vi "prototype UI_RESONANT.vi.REMOTE.vi"() -> ()   [LabVIEW 2012]
uses:
  GFG/GFG library.lvlib
  <vilib>/event_ctls.llb/lveventtype.ctl
  Custom Controls/scan mode main settings tab.ctl
  Custom Controls/file format type def.ctl
  Custom Controls/MAIN Image panel tab Control type def.ctl
  Custom Controls/Ch selector.ctl
  Custom Controls/advanced settings inner tab CTL.ctl
  Custom Controls/pixel resolution enum.ctl
  Custom Controls/display palette control.ctl
  Custom Controls/experiment type.ctl
  Custom Controls/Histogram tab.ctl
panel:
  in  "Objective":u16(ring) items=["10x Olympus", "20x Nikon", "30x Zeiss"]
  in  "x.voltage":dbl=0.9999999999999999 min=0.0 max=5.5 step=0.1
  in  "y.voltage":dbl=1.0 min=0.0 max=5.5 step=0.1
  in  "y.volt.offset":dbl=-0.2 step=0.1
  in  "x.volt.offset":dbl=-0.2 step=0.1
  in  "shutter":bool
  in  "x.pixels":i32=256 min=2 max=2048 step=2
  in  "clear prot":bool
  in  "timestamp.prot":bool
  in  "protocol.notes":string caption="notebook"
  in  "pos \nstore F":bool
  in  "pos \nstore E":bool
  in  "pos \nstore D":bool
  in  "pos \nstore C":bool
  in  "pos \nstore B":bool
  in  "pos \nstore A":bool
  out "String 10":string
  in  "pos \nrecall F":bool
  in  "pos \nrecall E":bool
  in  "pos \nrecall D":bool
  in  "pos \nrecall C":bool
  in  "pos \nrecall B":bool
  in  "pos \nrecall A":bool
  out "String 11":string
  in  "ref img\nOpen Files Button":bool
  in  "ref img\nstore F":bool
  in  "ref img\nstore E":bool
  in  "ref img\nstore D":bool
  in  "ref img\nstore C":bool
  in  "ref img\nstore B":bool
  in  "ref img\nstore A":bool
  out "String 17":string
  in  "ref img\nSave As Button":bool
  in  "Open All\nSettings":bool
  in  "step.size.z":u16(ring)=6 items=["  1"=1, "  2"=2, "  5"=5, " 10"=10, " 20"=20, " 50"=50, "100"=100]
  in  "Stage Stop":bool
  out "frame count":dbl(slide) scale=-1.0..430000.0
  in  "scan mode main settings":T1
  in  "x.correction":dbl(slide)=30.0 min=-100.0 max=100.0 step=1.0 scale=-100.0..100.0 scale format="%#_3g"
  in  "Start.Delay":dbl(slide)=220.0 min=1.0 max=320.0 step=1.0 scale=1.0..320.0 scale format="%#_3g"
  in  "pixel resolution":T2
  in  "ZOOM":dbl(slide)=1.0 min=1.0 max=3.0 step=0.1 scale=1.0..3.0 scale format="%_2g"
  in  "no. of frames to acquire":i32=10000 min=2 max=2147483646 step=2
  in  "x.fov":dbl caption="Field of view    x" format="%#_3p"
  in  "y.fov":dbl caption="y" format="%#_3p"
  out "frames.p.sec":dbl caption="frames/s" format="%#.2g"
  in  "resonant.correction.enable":bool
  out "pixels per line":i32=10000 min=2 max=2147483646 step=2
  out "lines per second":i32=10000 min=2 max=2147483646 step=2
  in  "linescan.y.pixels":i32=256 caption="Lines to display at once" min=2 max=2048 step=2
  in  "no. of lines to acquire":i32=10000 min=2 max=2147483646 step=2
  in  "experiment type":T3
  in  "experiment name":string
  in  "root.path":path=path "g:/"
  in  "file format":T4
  out "stack.duration":i32=10 caption="stack.duration (sec)" min=0 max=2147483646 step=2
  out "interpol XY":cluster{dbl[], "Best Exponential Fit":dbl[]}[](graph)
  in  "add":bool
  in  "clear all":bool
  in  "clear last":bool
  in  "move to z.stack.\nstart plane":bool
  in  "start z.stack":bool
  in  "frames.per.plane":i32=10000
  in  "z.spacing":dbl=1.0 caption="z.spacing (um)" min=0.1 step=0.1
  out "no of planes":i32=10 min=0 max=2147483646 step=2
  in  "piezo.mode":bool
  in  "frames.per.z.cycle":dbl=2.0 min=2.0 max=100.0 step=1.0
  in  "piezo.active":bool
  in  "Z UP":bool
  in  "Z DOWN":bool
  out "String 7":string
  in  "step.size.xy":u16(ring)=6 items=["  1"=1, "  2"=2, "  5"=5, " 10"=10, " 20"=20, " 50"=50, "100"=100]
  in  "Y UP":bool
  in  "X LEFT":bool
  in  "Y DOWN":bool
  in  "X RIGHT":bool
  out "String 6":string
  in  "setY":dbl caption="Z-Stepper" format="%#.1f"
  in  "setX":dbl caption="Z-Stepper" format="%#.1f"
  in  "setZ":dbl caption="set" format="%#.1f"
  out "String 4":string
  out "posZ":dbl caption="actual" format="%#.1f"
  out "posX":dbl caption="Z-Stepper" format="%#.1f"
  out "posY":dbl caption="Z-Stepper" format="%#.1f"
  out "String 3":string
  in  "XYZ stage settings slider tab":enum32{" "}(tab)
  in  "set Y to zero":bool
  in  "set X to zero":bool
  in  "set all to zero":bool
  in  "set Z to zero":bool
  out "String 9":string
  in  "reverse y":bool
  in  "reverse x":bool
  in  "reverse z":bool
  out "String 8":string
  in  "PIN Button stage settings":bool
  in  "QUIT":bool
  in  "Record":bool
  in  "FOCUS":bool
  in  "MAIN Image panels":T5
  out "Channel 1 large":T6(plugin-control)
  out "Channel 2 large":T6(plugin-control)
  out "Channel 3 large":T6(plugin-control)
  out "Channel 4 large":T6(plugin-control)
  out "Channel 1 small":T6(plugin-control)
  out "Channel 2 small":T6(plugin-control)
  out "Channel 4 small":T6(plugin-control)
  out "Channel 3 small":T6(plugin-control)
  in  "Blue Channel (Overlay)":T7 caption="B"
  in  "Green Channel (Overlay)":T7=enum."Ch 1" caption="G"
  in  "Red Channel (Overlay)":T7=enum."Ch 2" caption="R"
  out "RGB overlay":T6(plugin-control)
  out "ROI chart":sgl[][](graph)=[[54.570076, 54.556858]]
  in  "ROI channel":T7=enum."Ch 1" caption="Channel"
  out "ROI Image display":T6(plugin-control)
  in  "confirm line":bool
  in  "channel arb line scan":T7 caption="Channel"
  out "arb line scan display":T6(plugin-control)
  in  "Cancel":bool
  in  "hist/ref slider tab":enum32{" "}(tab)
  in  "PIN Button Hist/Ref":bool
  in  "Histograms tab":T8
  in  "auto scale\n      CH 1":bool=TRUE caption="auto scale 2"
  in  "Min Max Channel 1":cluster{dbl, dbl}(slide) scale=-33000.0..33000.0 scale format="%#_5g"
  out "Histogram 1":T9(graph)
  out "String 12":string
  in  "auto scale\n      CH 4":bool=TRUE caption="auto scale 2"
  in  "Min Max Channel 4":cluster{dbl, dbl}(slide) scale=-100.0..2047.0 scale format="%#_4g"
  out "Histogram 4":T9(graph)
  out "String 15":string
  in  "auto scale\n      CH 3":bool=TRUE caption="auto scale 2"
  in  "Min Max Channel 3":cluster{dbl, dbl}(slide) scale=-100.0..2047.0 scale format="%#_4g"
  out "Histogram 3":T9(graph)
  out "String 14":string
  in  "auto scale\n      CH 2":bool=TRUE caption="auto scale 2"
  in  "Min Max Channel 2":cluster{dbl, dbl}(slide) scale=-33000.0..33000.0 scale format="%#_4g"
  out "Histogram 2":T9(graph)
  out "String 13":string
  in  "avg type":u16(ring) items=["none", "group avg", "moving avg"]
  in  "avg of":i8=10 min=2 step=1
  in  "display palette":T10
  in  "laser power slider tab":enum32{""}(tab)
  in  "Laser Power":dbl(knob) min=0.0 max=100.0 step=0.5 scale=0.0..100.0 scale format="%3d"
  in  "PIN Button Pockels Control":bool
  in  "PMT slider tab":enum32{""}(tab)
  in  "PMT 2":u16(slide) max=1000 scale=0.0..1000.0
  in  "PMT 1":u16(slide) max=1250 scale=0.0..1000.0
  out "String 5":string
  in  "PMT 4":u16(slide) max=1000 scale=0.0..1000.0
  in  "PMT 3":u16(slide) max=1250 scale=0.0..1000.0
  out "String 18":string
  in  "PIN Button PMTs":bool
  in  "advanced settings slider tab":enum32{""}(tab)
  in  "advanced settings inner tab":T11
  in  "y.pixel.sz":dbl=1e-05 min=1e-09 max=1e-05 step=1e-07 format="%#_3p"
  in  "x.pixel.sz":dbl=1e-05 min=1e-09 max=1e-05 step=1e-07 format="%#_3p"
  in  "y.pixels":i32=256 caption="Y Resolution" min=2 max=2048 step=2
  in  "nomin.x.pixels":i32=256 caption="X resolution" min=2 max=2048 step=2
  in  "max.field.of.view\nresonant":dbl=300.0 format="%#_6p"
  in  "voltage.for\nmax.field.of.view\nresonant":dbl=5.0
  in  "max.field.of.view":dbl=300.0 format="%#_6p"
  in  "voltage.for\nmax.field.of.view":dbl=5.0
  in  "ai.active3":bool
  in  "ai.active2":bool
  in  "ai.active1":bool
  in  "ai.active0":bool caption="active?"
  in  "ai.range2":dbl=10.0 min=0.1 max=10.0 step=0.1
  in  "ai.range1":dbl=10.0 min=0.1 max=10.0 step=0.1
  out "ai.string3":string
  out "ai.string2":string
  out "ai.string1":string
  out "ai.string0":string caption="Analog Input"
  in  "ai.range0":dbl=10.0 caption="input range" min=0.1 max=10.0 step=0.1
  in  "ai.range3":dbl=10.0 min=0.1 max=10.0 step=0.1
  in  "external.start.trigger.enable":bool=TRUE caption="WAIT FOR TRIGGER"
  in  "pos  pockels cell PMT Data":dbl[][](array[numeric])=[[0.0, 0.0, 0.0, 0.0, 0.0, 0.0], [-200.0, 0.0, 0.0, 0.0, 0.0, 0.0]] caption="Data" format="%0.1f"
  in  "PIN Button Advanced Settings":bool
  in  "SCIENTIFICA Button":bool
  # "to zoom out press and hold Shift"
  # "current pos."
  # "go to pos."
  # "STORE positions"
  # "RECALL  positions"
  # "REFERENCE IMAGES"
  # "STORE"
  # "zig-zag (leaf scan)"
  # "planes"
  # "set zero"
  # "reverse \ndirection"
  # "1"
  # "2"
  # "3"
  # "4"
  # "Press and hold Ctrl to add multiple ROIs"
  # "This checkbox is only for starting the image acquisition using a TTL rising edge trigger from an external device. Don't tick this box unless an incoming trigger is wired up, otherwise the software may freeze. To reset, click QUIT and restart. If you want to send a trigger to an external device, just connect the ai.start.trigger.channel (e.g.PFI2, specified in settings.INI) to the external device, but leave the  checkbox above unticked."
  # "Z"
  # "laser"
  # "PMT1"
  # "PMT2"
  # "PMT3"
  # "PMT4"
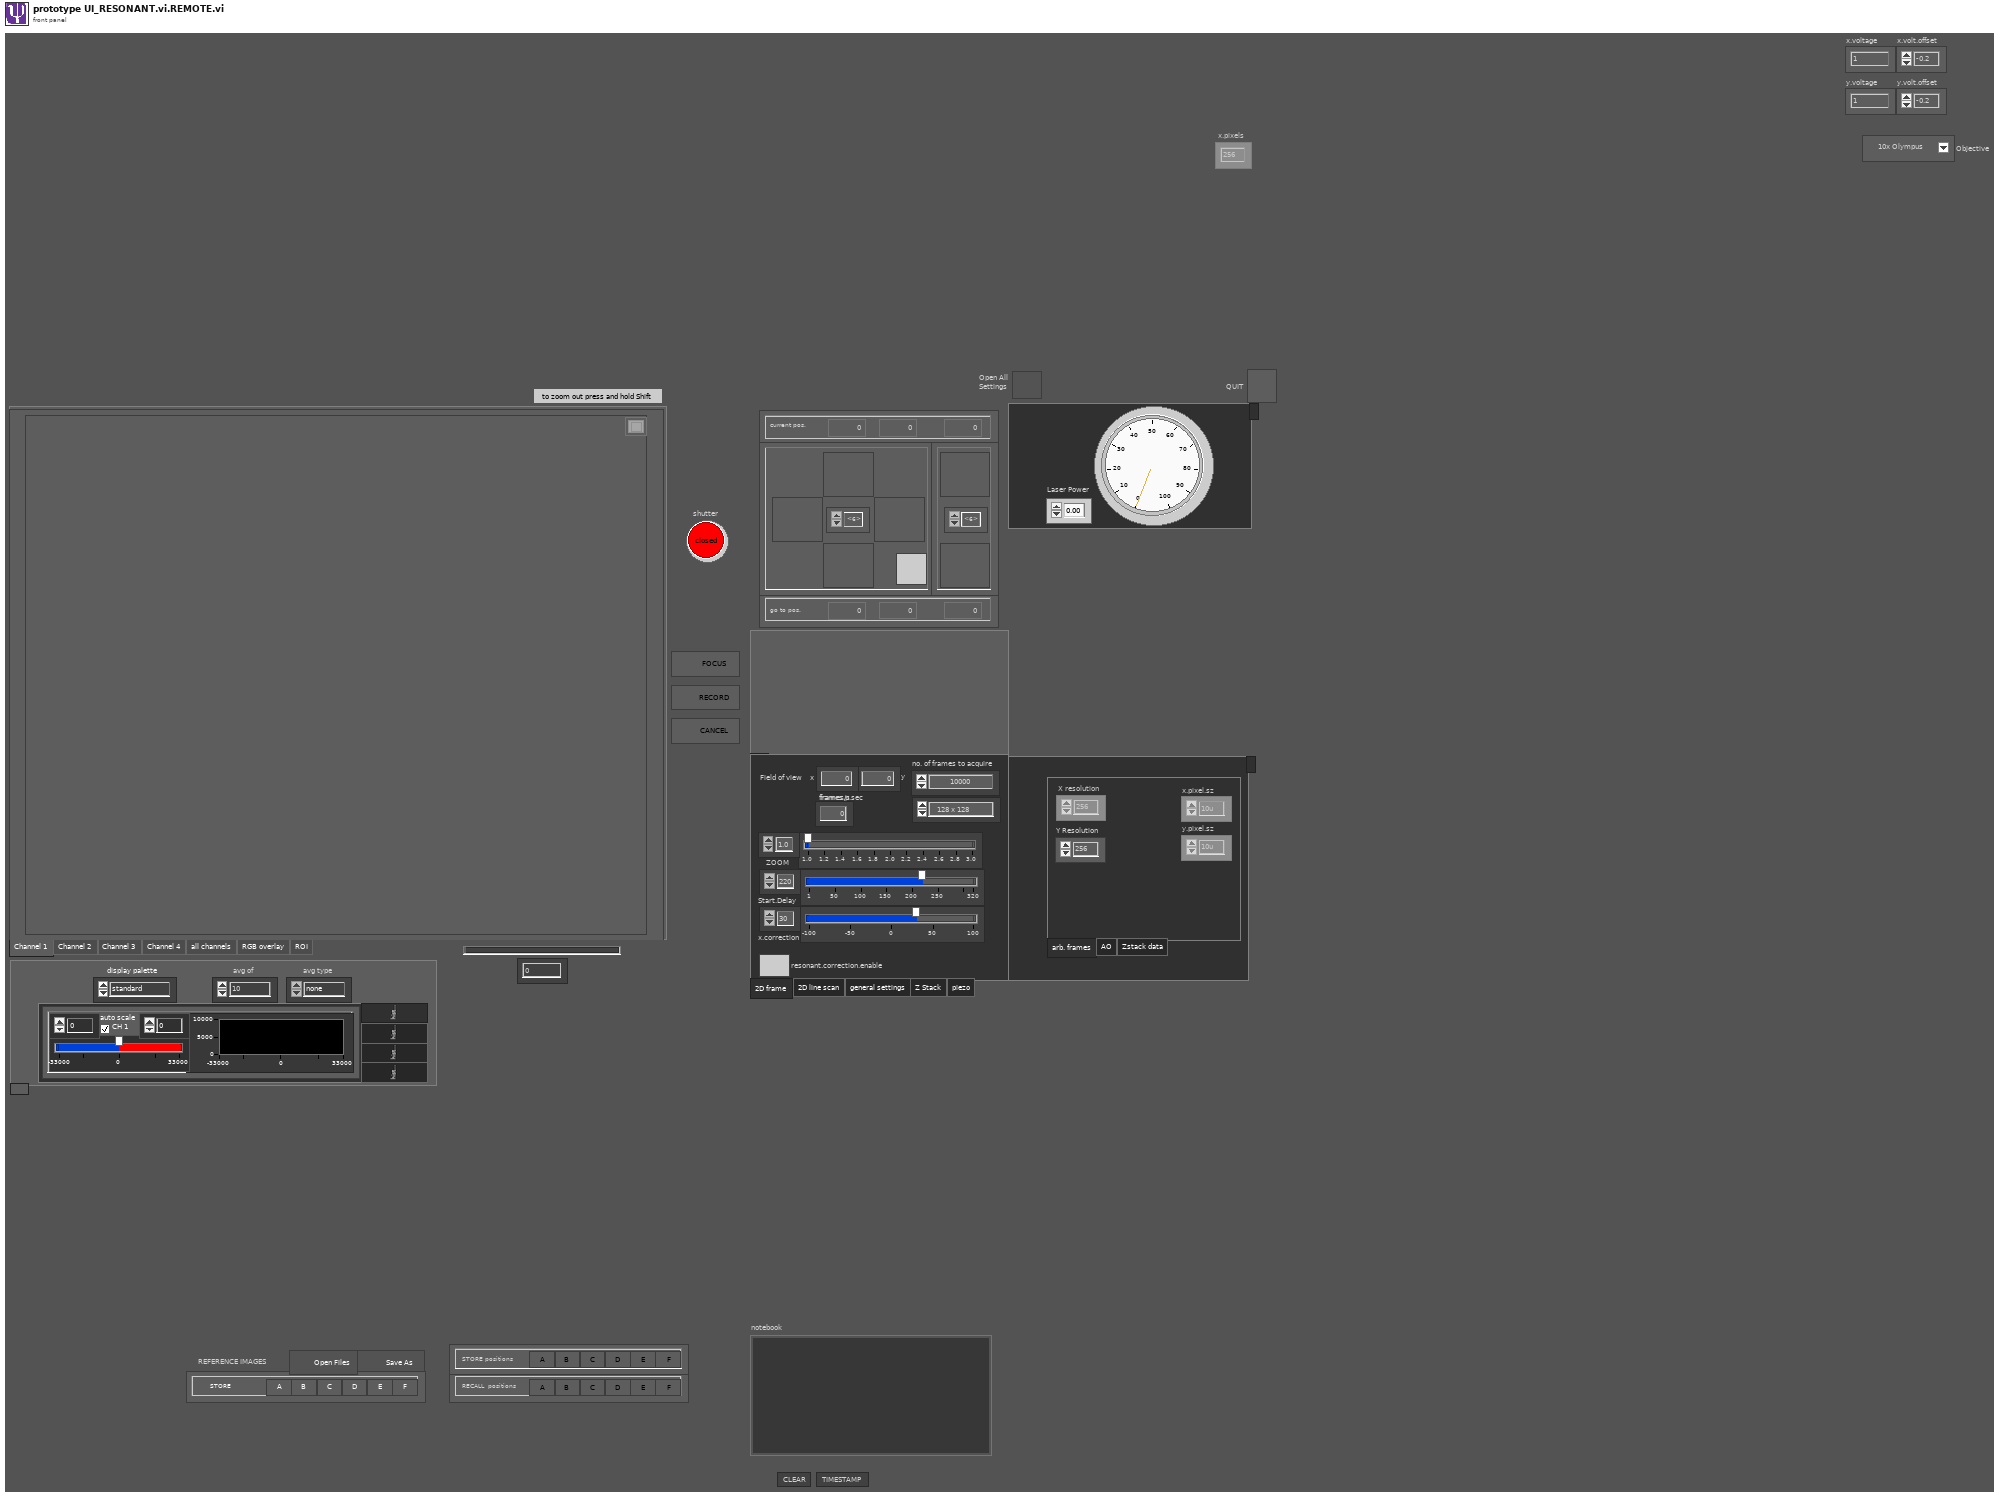
[diagram p1: front panel]
types:
  T1 = typedef "scan mode main settings tab.ctl" = enum32{"2D frame", "2D line scan", "general settings", "Z Stack", "piezo"}
  T2 = typedef "pixel resolution enum.ctl" = enum16{"   128 x 128", "   256 x 128", "   256 x 256", "   512 x 256", "   512 x 512", "  1024 x 512", "  1024 x 1024", "   arbitrary"}
  T3 = typedef "experiment type.ctl" = string
  T4 = typedef "file format type def.ctl" = enum16{"16bit raw", "32bit raw", "16bit multi-tiff (interleave)", "16bit multi-tiff (separate)", "16bit multi-tiff (stacked)", "32bit multi-tiff (interleave)", "32bit multi-tiff (separate)", "32bit multi-tiff (stacked)", "16bit tiff series (interleave)", "16bit tiff series (separate)", "16bit tiff series (stacked)", "32bit tiff series (interleave)", "32bit tiff series (separate)", "32bit tiff series (stacked)"}
  T5 = typedef "MAIN Image panel tab Control type def.ctl" = enum32{"Channel 1", "Channel 2", "Channel 3", "Channel 4", "all channels", "RGB overlay", "ROI", "arbitrary line scan"}
  T6 = typedef "IMAQ Image.ctl" = refnum<image>
  T7 = typedef "Ch selector.ctl" = enum16{"none", "Ch 1", "Ch 2", "Ch 3", "Ch 4", "Ch 5"}
  T8 = typedef "Histogram tab.ctl" = enum32{"hist Ch 1", "hist Ch 4", "hist Ch 3", "hist Ch 2"}
  T9 = cluster{"Starting Value":sgl, "Incremental Value":sgl, "Histogram":u32[]}
  T10 = typedef "display palette control.ctl" = enum16{"standard", "high clipping red", "low clipping blue", "high and low clipping"}
  T11 = typedef "advanced settings inner tab CTL.ctl" = enum32{"arb. frames", "AO", "AI", "channels", "trigger", "Zstack data"}
  T12 = enum8{"Enabled", "Disabled", "Disabled and Grayed Out"}
  T13 = typedef "Image Type" = u32
  T14 = cluster{refnum<vi>, refnum<vi>, refnum<vi>, refnum<vi>, refnum<vi>, refnum<vi>, refnum<vi>, refnum<vi>, refnum<vi>, refnum<vi>, refnum<vi>}
  T15 = cluster{"New Image":T6, "New Image":T6, "New Image":T6, "New Image":T6, "New Image":T6, "New Image":T6, "New Image":T6, "New Image":T6, "New Image":T6, "New Image":T6, "New Image":T6}
  T16 = typedef "lveventtype.ctl" = enum32{"Null", "Timeout", "Annotation Menu Selection", "Annotation Menu Selection?", "App Instance Close", "App Instance Close?", "Autoscale Range Change", "Cell Edit", "Cell Edit?", "Cursor Grab", "Cursor Grab?", "Cursor Menu Selection", "Cursor Menu Selection?", "Cursor Move", "Cursor Release", "Data Change", "Direction Change", "Display State Change", "Drag Ended", "Drag Enter", "Drag Leave", "Drag Over", "Drag Source Update", "Drag Starting", "Drag Starting?", "Drop", "Exec State Change", "Key Down", "Key Down?", "Key Repeat", "Key Repeat?", "Key Up", "Listbox Double Click", "Menu Activation?", "Menu Selection (App)", "Menu Selection? (App)", "Menu Selection (User)", "Mouse Down", "Mouse Down?", "Mouse Enter", "Mouse Leave", "Mouse Move", "Mouse Up", "NI Security User Change (App)", "Pane Size", "Panel Close", "Panel Close?", "Panel Resize", "Plot Attribute Change", "Scale Range Change", "Shortcut Menu Activation?", "Shortcut Menu Selection (App)", "Shortcut Menu Selection? (App)", "Shortcut Menu Selection (User)", "Tree Double Click", "Tree Drag", "Tree Drag?", "Tree Drop", "Tree Drop?", "Tree Item Close", "Tree Item Close?", "Tree Item Open", "Tree Item Open?", "Value Change"}
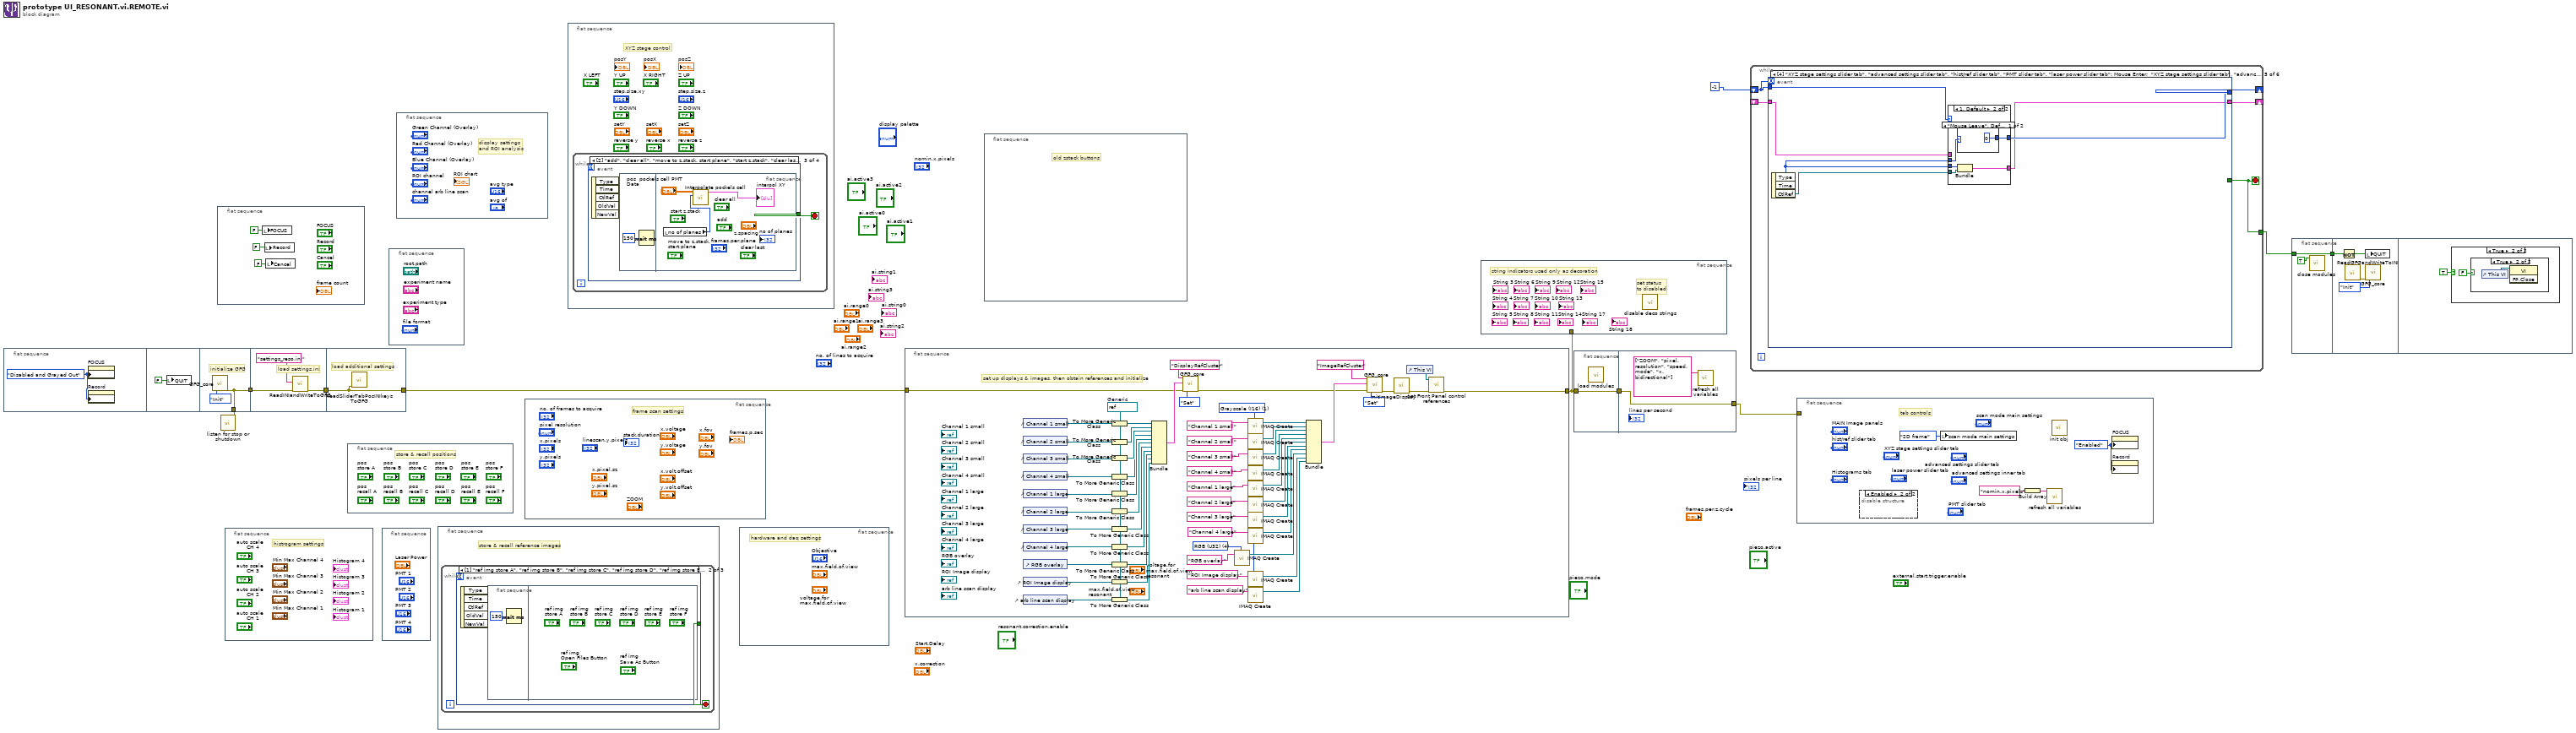
[diagram p0: block diagram]
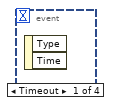
[diagram p2: hidden frame]
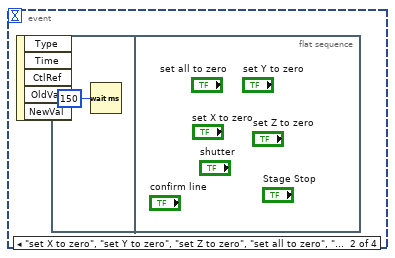
[diagram p3: hidden frame]
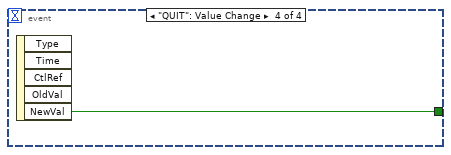
[diagram p4: hidden frame]
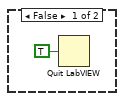
[diagram p5: hidden frame]
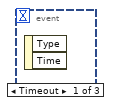
[diagram p7: hidden frame]
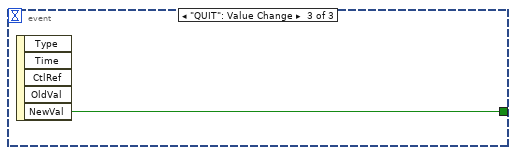
[diagram p8: hidden frame]
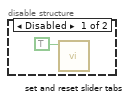
[diagram p9: hidden frame]
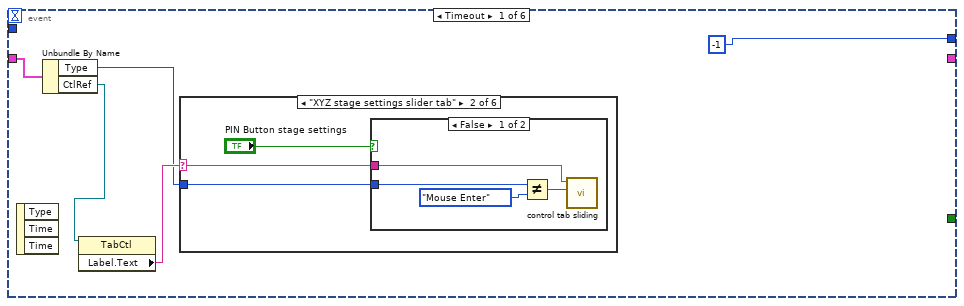
[diagram p10: hidden frame]
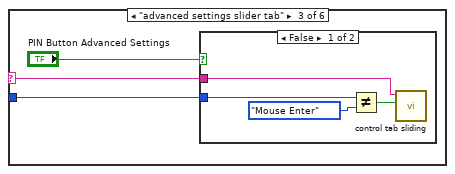
[diagram p13: hidden frame]
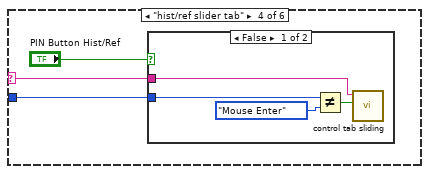
[diagram p15: hidden frame]
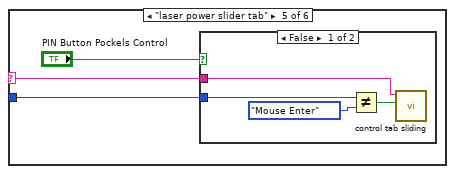
[diagram p17: hidden frame]
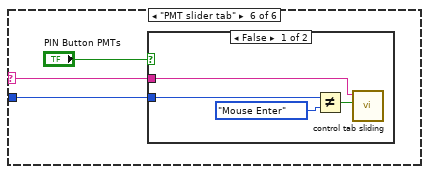
[diagram p19: hidden frame]
diagram:
  n1 = flat-sequence {
    tunnel: [w13] -> w10
    tunnel: [w13] -> w9
    tunnel: w10 -> [w17]
    tunnel: [w16] -> w3
    tunnel: [w18] -> w6
    tunnel: w3 -> [w18]
    frame #0 {
      w11 = T12."Disabled and Grayed Out" ("Disabled")
      n2 = property on="FOCUS" class="Bool (strict)"("DisabledEnum"=w11) -> ()  [unwired: 2 in, 2 out]
      n3 = property on="Record" class="Bool (strict)"("DisabledEnum"=w11) -> ()  [unwired: 2 in, 2 out]
    }
    frame #1 {
      n4 = local write "QUIT"(FALSE ("QUIT")) -> ()
    }
    frame #2 {
      # "initialize GFG"
      n5 = call "GFG_core.vi"("Action"=enum16{"Init", "Set", "Get"}."Init") -> ("error out"=w13:errorcluster)  [unwired: 12 in, 6 out]
    }
    frame #3 {
      # "load settings.ini"
      n6 = call "ReadINIandWriteToGFG.vi"("error in (no error)"=w17, "name or relative path"="settings_reso.ini") -> ("error out"=w16:errorcluster)  [unwired: 9 in]
    }
    frame #4 {
      # "load additional settings"
      n7 = call "ReadSliderTabPosINIkeysToGFG.vi"("error in (no error)"=w18) -> ()  [unwired: 11 in]
    }
  }
  n8 = flat-sequence {
    frame #0 {
      n9 = local write "FOCUS"(FALSE ("FOCUS")) -> ()
      n10 = local write "Record"(FALSE ("Record")) -> ()
      n11 = local write "Cancel"(FALSE ("Cancel")) -> ()
    }
  }
  n12 = call "listen for stop or shutdown.vi"("error in (no error)"=w9) -> ()  [unwired: 9 in, 2 out]
  n13 = flat-sequence {
    frame #0 {
      # "histrogram settings"
    }
  }
  n14 = flat-sequence {
    frame #0 {
      # "store & recall positions"
    }
  }
  n15 = flat-sequence {
    frame #0 {
    }
  }
  n16 = flat-sequence {
    frame #0 {
    }
  }
  n17 = flat-sequence {
    frame #0 {
      # "display settings\nand ROI analysis"
    }
  }
  n18 = flat-sequence {
    frame #0 {
      # "store & recall reference images"
      n19 = while {
        stop <- w22 stop-if-true
        n20 = event shown="[1] \"ref img store A\", \"ref img store B\", \"ref img store C\", \"ref img store D\", \"ref img store E\", \"ref img store F\", \"ref img Save As Button\", \"ref img Open Files Button\": Value Change" {
          selector: _ -> [_ _ _]
          dyn-events: _ -> [_ _ _]
          timeout: _ -> [_ _ _]
          tunnel: [_ _ w24] -> w22
          event Timeout {
            n21 = event-data() -> ()  [unwired: 1 in, 2 out]
          }
          event "ref img\nstore A", "ref img\nstore B", "ref img\nstore C", "ref img\nstore D", "ref img\nstore E", "ref img\nstore F", "ref img\nSave As Button", "ref img\nOpen Files Button": Value Change {
            n22 = event-data() -> ()  [unwired: 1 in, 5 out]
            n23 = flat-sequence {
              frame #0 {
                n24 = Wait (ms)(milliseconds to wait=u32 150) -> ()  [unwired: 1 out]
              }
              frame #1 {
              }
            }
          }
          event "QUIT": Value Change {
            n25 = event-data() -> ("NewVal"=w24:bool)  [unwired: 1 in, 4 out]
          }
        }
      }
    }
  }
  n26 = flat-sequence {
    frame #0 {
      # "frame scan settings"
    }
  }
  n27 = flat-sequence {
    frame #0 {
      # "XYZ stage control"
      n28 = while {
        stop <- w25 stop-if-true
        n29 = event shown="[2] \"add\", \"clear all\", \"move to z.stack. start plane\", \"start z.stack\", \"clear last\", \"z.spacing\", \"frames.per.plane\", \"no of planes\", \"pos  pockels cell PMT Data\": Value Change" {
          selector: _ -> [_ _ _ _]
          dyn-events: _ -> [_ _ _ _]
          timeout: _ -> [_ _ _ _]
          tunnel: [_ _ _ w31] -> w25
          event Timeout {
            n30 = event-data() -> ()  [unwired: 1 in, 2 out]
          }
          event "set X to zero", "set Y to zero", "set Z to zero", "set all to zero", "confirm line", "Stage Stop": Value Change {
            n31 = event-data() -> ()  [unwired: 1 in, 5 out]
            n32 = flat-sequence {
              frame #0 {
                n33 = Wait (ms)(milliseconds to wait=u32 150) -> ()  [unwired: 1 out]
              }
              frame #1 {
              }
            }
          }
          event "add", "clear all", "move to z.stack.\nstart plane", "start z.stack", "clear last", "z.spacing", "frames.per.plane", "no of planes", "pos  pockels cell PMT Data": Value Change {
            n34 = event-data() -> ()  [unwired: 1 in, 5 out]
            n35 = flat-sequence {
              frame #0 {
                n36 = Wait (ms)(milliseconds to wait=u32 150) -> ()  [unwired: 1 out]
              }
              frame #1 {
                n37 = local read "no of planes"() -> (w28:i32)
                n38 = call "Interpolate pockels cell.vi"("nr of planes"=w28, "Data"="pos  pockels cell PMT Data") -> ("Raw Data and Interpolated Data"=→"interpol XY":cluster{dbl[], "Best Exponential Fit":dbl[]}[])  [unwired: 8 in, 1 out]
              }
            }
          }
          event "QUIT": Value Change {
            n39 = event-data() -> ("NewVal"=w31:bool)  [unwired: 1 in, 4 out]
          }
        }
      }
    }
  }
  n40 = flat-sequence {
    frame #0 {
      # "hardware and daq settings"
    }
  }
  n41 = flat-sequence {
    tunnel: [w46] -> w7
    tunnel: w6 -> [w45]
    frame #0 {
      w33 = T13 4 items=["Grayscale (U8)", "Grayscale (I16)", "Grayscale (SGL)", "Complex (CSG)", "RGB (U32)", "HSL (U32)", "RGB (U64)", "Grayscale (U16)"] ("Image Type")
      w32 = T13 1 items=["Grayscale (U8)", "Grayscale (I16)", "Grayscale (SGL)", "Complex (CSG)", "RGB (U32)", "HSL (U32)", "RGB (U64)", "Grayscale (U16)"] ("Image Type")
      w76 = refnum<vi> refnum  # Generic
      # "set up displays & images, then obtain references and initialize"
      n42 = control-ref of="Channel 1 small"() -> (w44:refnum<vi>)
      n43 = control-ref of="Channel 2 small"() -> (w43:refnum<vi>)
      n44 = control-ref of="Channel 3 small"() -> (w42:refnum<vi>)
      n45 = control-ref of="Channel 4 small"() -> (w41:refnum<vi>)
      n46 = control-ref of="Channel 1 large"() -> (w40:refnum<vi>)
      n47 = control-ref of="Channel 2 large"() -> (w39:refnum<vi>)
      n48 = control-ref of="Channel 3 large"() -> (w38:refnum<vi>)
      n49 = control-ref of="Channel 4 large"() -> (w37:refnum<vi>)
      n50 = control-ref of="RGB overlay"() -> (w36:refnum<vi>)
      n51 = control-ref of="ROI Image display"() -> (w35:refnum<vi>)
      n52 = control-ref of="arb line scan display"() -> (w34:refnum<vi>)
      n53 = To More Generic Class(target class=w76, reference=w44) -> (generic class reference=w87:refnum<vi>)
      n54 = To More Generic Class(target class=w76, reference=w43) -> (generic class reference=w80:refnum<vi>)
      n55 = To More Generic Class(target class=w76, reference=w42) -> (generic class reference=w79:refnum<vi>)
      n56 = To More Generic Class(target class=w76, reference=w41) -> (generic class reference=w78:refnum<vi>)
      n57 = To More Generic Class(target class=w76, reference=w40) -> (generic class reference=w77:refnum<vi>)
      n58 = To More Generic Class(target class=w76, reference=w39) -> (generic class reference=w86:refnum<vi>)
      n59 = To More Generic Class(target class=w76, reference=w38) -> (generic class reference=w85:refnum<vi>)
      n60 = To More Generic Class(target class=w76, reference=w37) -> (generic class reference=w84:refnum<vi>)
      n61 = To More Generic Class(target class=w76, reference=w36) -> (generic class reference=w83:refnum<vi>)
      n62 = To More Generic Class(target class=w76, reference=w35) -> (generic class reference=w82:refnum<vi>)
      n63 = To More Generic Class(target class=w76, reference=w34) -> (generic class reference=w81:refnum<vi>)
      n64 = Bundle(w87, w80, w79, w78, w77, w86, w85, w84, w83, w82, w81) -> (w90:T14)  [unwired: 1 in]
      n65 = call "GFG_core.vi"("Variable Name in"="DisplayRefCluster", "Variant in"=w90, "error in (no error)"=w45, "Action"=enum16{"Init", "Set", "Get"}."Set") -> ("error out"=w50:errorcluster)  [unwired: 9 in, 6 out]
      n66 = call "IMAQ Create"("Image Name"="RGB overlay", "Image Type"=w33) -> ("New Image"=w70:T6)  [unwired: 3 in, 1 out]
      n67 = call "IMAQ Create"("Image Name"="Channel 1 small", "Image Type"=w32) -> ("New Image"=w62:T6)  [unwired: 3 in, 1 out]
      n68 = call "IMAQ Create"("Image Name"="Channel 2 small", "Image Type"=w32) -> ("New Image"=w63:T6)  [unwired: 3 in, 1 out]
      n69 = call "IMAQ Create"("Image Name"="Channel 3 small", "Image Type"=w32) -> ("New Image"=w64:T6)  [unwired: 3 in, 1 out]
      n70 = call "IMAQ Create"("Image Name"="Channel 4 small", "Image Type"=w32) -> ("New Image"=w65:T6)  [unwired: 3 in, 1 out]
      n71 = call "IMAQ Create"("Image Name"="Channel 1 large", "Image Type"=w32) -> ("New Image"=w66:T6)  [unwired: 3 in, 1 out]
      n72 = call "IMAQ Create"("Image Name"="Channel 2 large", "Image Type"=w32) -> ("New Image"=w67:T6)  [unwired: 3 in, 1 out]
      n73 = call "IMAQ Create"("Image Name"="Channel 3 large", "Image Type"=w32) -> ("New Image"=w68:T6)  [unwired: 3 in, 1 out]
      n74 = call "IMAQ Create"("Image Name"="Channel 4 large", "Image Type"=w32) -> ("New Image"=w69:T6)  [unwired: 3 in, 1 out]
      n75 = call "IMAQ Create"("Image Name"="ROI Image display", "Image Type"=w32) -> ("New Image"=w71:T6)  [unwired: 3 in, 1 out]
      n76 = call "IMAQ Create"("Image Name"="arb line scan display", "Image Type"=w32) -> ("New Image"=w72:T6)  [unwired: 3 in, 1 out]
      n77 = Bundle("New Image"=w62, "New Image"=w63, "New Image"=w64, "New Image"=w65, "New Image"=w66, "New Image"=w67, "New Image"=w68, "New Image"=w69, "New Image"=w70, "New Image"=w71, "New Image"=w72) -> (w74:T15)  [unwired: 1 in]
      n78 = call "GFG_core.vi"("Variable Name in"="ImageRefCluster", "Variant in"=w74, "error in (no error)"=w50, "Action"=enum16{"Init", "Set", "Get"}."Set") -> ("error out"=w49:errorcluster)  [unwired: 9 in, 6 out]
      n79 = call "InitImageDisplay.vi"("error in (no error)"=w49) -> ("error out"=w48:errorcluster)  [unwired: 10 in]
      n80 = control-ref of="This VI"() -> (w47:refnum<vi>)
      n81 = call "get Front Panel control references.vi"("error in (no error)"=w48, "Main VI"=w47) -> ("error out"=w46:errorcluster)  [unwired: 9 in]
    }
  }
  n82 = flat-sequence {
    frame #0 {
      # "old zstack buttons"
    }
  }
  n83 = flat-sequence {
    tunnel: w7 -> [_]
    frame #0 {
      # "set status\nto disabled"
      # "string indicators used only as decoration"
      n84 = call "disable deco strings.vi"() -> ()  [unwired: 11 in, 1 out]
    }
  }
  n85 = flat-sequence {
    tunnel: w7 -> [w91]
    tunnel: [w91] -> w2
    tunnel: [w93] -> w1
    tunnel: w2 -> [w93]
    frame #0 {
      n86 = call "load modules.vi"() -> ()  [unwired: 12 in]
    }
    frame #1 {
      n87 = call "refresh all variables.vi"("All Variable Names"=string[] ["ZOOM", "pixel.resolution", "speed.mode", "x.bidirectional"] ("Variables Names In")) -> ()  [unwired: 11 in]
    }
  }
  n88 = while {
    tunnel: [w98] -> w8
    shift-right: [w97] -> _
    shift-left: _ -> [w95]
    shift-right: [w96] -> _
    shift-left: -1 -> [w94]
    stop <- w98 stop-if-true
    n89 = event shown="[4] \"XYZ stage settings slider tab\", \"advanced settings slider tab\", \"hist/ref slider tab\", \"PMT slider tab\", \"laser power slider tab\": Mouse Enter;  \"XYZ stage settings slider tab\", \"advanced settings slider tab\", \"hist/ref slider tab\", \"PMT slider tab\", \"laser power slider tab\": Mouse Leave" {
      selector: _ -> [_ _ _ _ _ _]
      dyn-events: _ -> [_ _ _ _ _ _]
      timeout: w94 -> [_ _ _ _ _ _]
      tunnel: [_ _ "QUIT" _ _ _] -> w98
      tunnel: [_ _ _ _ w155 _] -> w97
      tunnel: [-1 w139 w150 w152 w159 w169] -> w96
      tunnel: w95 -> [w103 _ _ _ w154 _]
      tunnel: w94 -> [_ w139 w150 w152 w158 w169]
      event Timeout {
        n90 = event-data() -> ()  [unwired: 1 in, 3 out]
        n91 = Unbundle By Name(w103) -> ("Type"=w100:T16, "CtlRef"=w102:refnum<vi>)
        n92 = property class="TabCtl"(reference=w102) -> ("Label.Text"=w101:string)  [unwired: 1 in, 2 out]
        n93 = case shown="\"XYZ stage settings slider tab\"" w101 {
          selector: w101 -> [_ w105 w111 w120 w125 w134]
          tunnel: w100 -> [_ w104 w112 w118 w126 w133]
          frame "False", Default {
          }
          frame "XYZ stage settings slider tab" {
            n94 = case shown="False" "PIN Button stage settings" {
              tunnel: w105 -> [w110 _]
              tunnel: w104 -> [w109 _]
              frame False {
                n95 = Not Equal?(x=w109, y=lveventtype."Mouse Enter" ("Type")) -> (x != y?=w108:bool)
                n96 = call "control tab sliding.vi"("close(T)/open(F)"=w108, "String"=w110) -> ()  [unwired: 10 in]
              }
              frame True {
              }
            }
          }
          frame "advanced settings slider tab" {
            n97 = case shown="False" "PIN Button Advanced Settings" {
              tunnel: w111 -> [w117 _]
              tunnel: w112 -> [w116 _]
              frame False {
                n98 = Not Equal?(x=w116, y=lveventtype."Mouse Enter" ("Type")) -> (x != y?=w115:bool)
                n99 = call "control tab sliding.vi"("close(T)/open(F)"=w115, "String"=w117) -> ()  [unwired: 10 in]
              }
              frame True {
              }
            }
          }
          frame "hist/ref slider tab" {
            n100 = case shown="False" "PIN Button Hist/Ref" {
              tunnel: w120 -> [w124 _]
              tunnel: w118 -> [w123 _]
              frame False {
                n101 = Not Equal?(x=w123, y=lveventtype."Mouse Enter" ("Type")) -> (x != y?=w122:bool)
                n102 = call "control tab sliding.vi"("close(T)/open(F)"=w122, "String"=w124) -> ()  [unwired: 10 in]
              }
              frame True {
              }
            }
          }
          frame "laser power slider tab" {
            n103 = case shown="False" "PIN Button Pockels Control" {
              tunnel: w125 -> [w131 _]
              tunnel: w126 -> [w130 _]
              frame False {
                n104 = Not Equal?(x=w130, y=lveventtype."Mouse Enter" ("Type")) -> (x != y?=w129:bool)
                n105 = call "control tab sliding.vi"("close(T)/open(F)"=w129, "String"=w131) -> ()  [unwired: 10 in]
              }
              frame True {
              }
            }
          }
          frame "PMT slider tab" {
            n106 = case shown="False" "PIN Button PMTs" {
              tunnel: w134 -> [w138 _]
              tunnel: w133 -> [w137 _]
              frame False {
                n107 = Not Equal?(x=w137, y=lveventtype."Mouse Enter" ("Type")) -> (x != y?=w136:bool)
                n108 = call "control tab sliding.vi"("close(T)/open(F)"=w136, "String"=w138) -> ()  [unwired: 10 in]
              }
              frame True {
              }
            }
          }
        }
      }
      event "Open All\nSettings": Value Change {
        n109 = event-data() -> ()  [unwired: 1 in, 5 out]
        n110 = case shown="True" "Open All\nSettings" {
          frame False {
            n111 = call "slider tabs open.vi"("close(T)/open(F)"=TRUE) -> ()  [unwired: 11 in]
          }
          frame True {
            n112 = call "slider tabs open.vi"("close(T)/open(F)"=FALSE) -> ()  [unwired: 11 in]
          }
        }
      }
      event "QUIT": Value Change {
        n113 = event-data() -> ()  [unwired: 1 in, 5 out]
        n114 = call "getVIname.vi"() -> ("VI name"=w149:string)  [unwired: 19 in]
        n115 = call "SendShutdownCommand.vi"("Source VI"=w149) -> ()  [unwired: 11 in]
        n116 = call "GFG_core.vi"("Variable Name in"="shutter", "Variant in"=FALSE ("QUIT"), "Action"=enum16{"Init", "Set", "Get"}."Set") -> ()  [unwired: 10 in, 7 out]
        n117 = call "GFG_core.vi"("Variable Name in"="Cancel", "Variant in"=FALSE ("QUIT"), "Action"=enum16{"Init", "Set", "Get"}."Set") -> ()  [unwired: 10 in, 7 out]
      }
      event "SCIENTIFICA Button": Value Change {
        n118 = event-data() -> ()  [unwired: 1 in, 5 out]
        n119 = call <vilib>:"Open URL in Default Browser (string).vi"("URL"="http://www.scientifica.uk.com/") -> ()  [unwired: 5 in, 2 out]
      }
      event "XYZ stage settings slider tab", "advanced settings slider tab", "hist/ref slider tab", "PMT slider tab", "laser power slider tab": Mouse Enter; "XYZ stage settings slider tab", "advanced settings slider tab", "hist/ref slider tab", "PMT slider tab", "laser power slider tab": Mouse Leave {
        n120 = event-data() -> ("Type"=w157:T16, "CtlRef"=w156:refnum<vi>)  [unwired: 1 in, 1 out]
        n121 = case shown="1, Default" w158 {
          tunnel: [0 w166] -> w159
          tunnel: w157 -> [_ w165]
          tunnel: w157 -> [_ w164]
          tunnel: w156 -> [_ w163]
          tunnel: [w160 w162] -> w155
          tunnel: w154 -> [w160 _]
          frame 0 {
          }
          frame 1, Default {
            n122 = case shown="\"Mouse Leave\", Default" w165 {
              tunnel: [0 150] -> w166
              frame "Mouse Leave", Default {
              }
              frame "Mouse Enter" {
              }
            }
            n123 = Bundle("Type"=w164, "CtlRef"=w163) -> (w162:cluster{"Type":T16, "CtlRef":refnum<vi>})  [unwired: 1 in]
          }
        }
      }
      event "clear prot", "timestamp.prot", "protocol.notes": Value Change {
        n124 = event-data() -> ("CtlRef"=w173:refnum<vi>)  [unwired: 1 in, 4 out]
        n125 = property class="Ctl"(reference=w173) -> ("Label.Text"=w172:string)  [unwired: 1 in, 2 out]
        n126 = case shown="\"clear prot\"" w172 {
          tunnel: "protocol.notes" -> [w174 w176 _]
          tunnel: [w174 w175 ""] -> w170
          frame "Null", Default {
          }
          frame "timestamp.prot" {
            n127 = Get Date/Time In Seconds() -> (seconds since 1Jan1904=w179:timestamp)
            n128 = Format Date/Time String(time format string (%c)="%Y-%m-%d %H:%M:%S%2u", seconds (now)=w179) -> (date/time string=w177:string)  [unwired: 1 in]
            n129 = Concatenate Strings(w176, "\n##################\n" ("string"), w177) -> (w175:string)
          }
          frame "clear prot" {
          }
        }
        n130 = local write "protocol.notes"(w170) -> ()
      }
    }
  }
  n131 = flat-sequence {
    tunnel: w1 -> [_]
    frame #0 {
      w182 = T12."Enabled" ("Disabled")
      # "tab controls"
      n132 = disable-structure shown="Enabled" {
        frame Disabled {
          n133 = call "set and reset slider tabs.vi"("Set(T)/Reset(F)"=TRUE) -> ()  [unwired: 11 in]
        }
        frame Enabled {
        }
      }
      n134 = local write "scan mode main settings"(scan_mode_main_settings_tab."2D frame" ("scan mode main settings")) -> ()
      n135 = Build Array("nomin.x.pixels" ("Variable Name in")) -> (w185:string[])
      n136 = call "refresh all variables.vi"("All Variable Names"=w185) -> ()  [unwired: 11 in]
      n137 = call "init obj.vi"() -> ()  [unwired: 12 in]
      n138 = property on="FOCUS" class="Bool (strict)"("DisabledEnum"=w182) -> ()  [unwired: 2 in, 2 out]
      n139 = property on="Record" class="Bool (strict)"("DisabledEnum"=w182) -> ()  [unwired: 2 in, 2 out]
    }
  }
  n140 = flat-sequence {
    tunnel: w8 -> [w188]
    tunnel: [w188] -> w4
    tunnel: w4 -> [w189]
    frame #0 {
      n141 = call "close modules.vi"("close FP?"=TRUE) -> ()  [unwired: 11 in]
    }
    frame #1 {
      n142 = Not(x=w189) -> (.not. x?=w190:bool)
      n143 = call "ReadGFGandWriteToINI.vi"() -> ("error out"=w191:errorcluster)  [unwired: 11 in]
      n144 = local write "QUIT"(w190) -> ()
      n145 = call "GFG_core.vi"("error in (no error)"=w191, "Action"=enum16{"Init", "Set", "Get"}."Init") -> ()  [unwired: 11 in, 7 out]
    }
    frame #2 {
      n146 = case shown="True" TRUE {
        frame False {
          n147 = Quit LabVIEW(quit? (T)=TRUE) -> ()
        }
        frame True {
          n148 = case shown="True" FALSE {
            frame False {
            }
            frame True {
              n149 = control-ref of="This VI"() -> (w196:refnum<vi>)
              n150 = invoke class="VI" method="FP.Close"(reference=w196) -> ()  [unwired: 2 in, 3 out]
            }
          }
        }
      }
    }
  }
